vi "CRYGraph Property Window Result.vi"(8 "Tab Name":string, 9 "Graph VI Ref":refnum<vi>) -> ()   [LabVIEW 2013]
uses:
  Control/CRYResult Property.ctl
panel:
  in  "Redraw":bool
  in  "Draw":bool
  in  "Result Property":T1={"Show Limits"=FALSE, "Show Yield"=FALSE, "Pass/Fail"=FALSE, "Notation"=0, "Digits"=0, "Precision"=0, "Hide Traling Zeros"=FALSE, "Show vertical scroll bar"=FALSE, "Show horizontal scroll bar"=FALSE, "True"="NO ELECTRICAL SIGNAL DETECTED!\nCheck wiring and connections.", "False"="NO ELECTRICAL SIGNAL DETECTED!\nCheck wiring and connections.", "Font Size"=0, "Overall/Optional"=0} {"Precision" items=["Digits of precision", "Significant digits"]}
  in  "OK":bool
  in  "Result Tab":enum32{"Title", "Format"}(tab)
  in  "Title Name":string
  in  "Show vertical scroll bar":bool
  in  "Show horizontal scroll bar":bool
  in  "Overall/Optional":u16(slide) caption="Notation"
  in  "Font Size":u16
  in  "False":string
  in  "True":string
  in  "Hide Traling Zeros":bool caption="Hide Trailing Zeros"
  in  "PrecisionType":u16(ring) caption="Precision" items=["Digitals of precision", "Significant digits "]
  in  "Digits":u16
  in  "Notation":u16(slide)
  in  "Pass/Fail":bool
  in  "Show Yield":bool
  in  "Show Limits":bool
  out "Number Format":bool
  out "Settings":bool
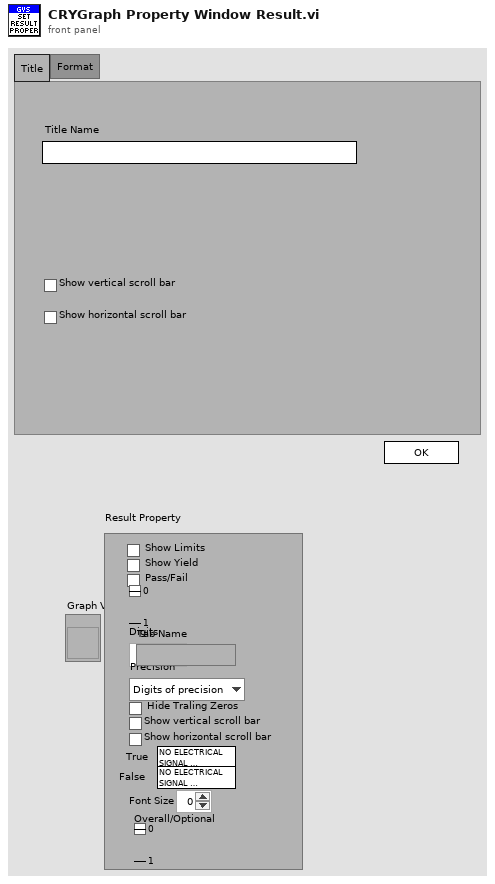
[diagram p1: front panel]
types:
  T1 = typedef "CRYResult Property.ctl" = cluster{"Show Limits":bool, "Show Yield":bool, "Pass/Fail":bool, "Notation":u16, "Digits":u16, "Precision":u16, "Hide Traling Zeros":bool, "Show vertical scroll bar":bool, "Show horizontal scroll bar":bool, "True":string, "False":string, "Font Size":u16, "Overall/Optional":u16}
  T2 = enum32{"Page Enabled", "Page Disabled", "Page Disabled & Grayed"}
  T3 = enum8{"Enabled", "Disabled", "Disabled and Grayed Out"}
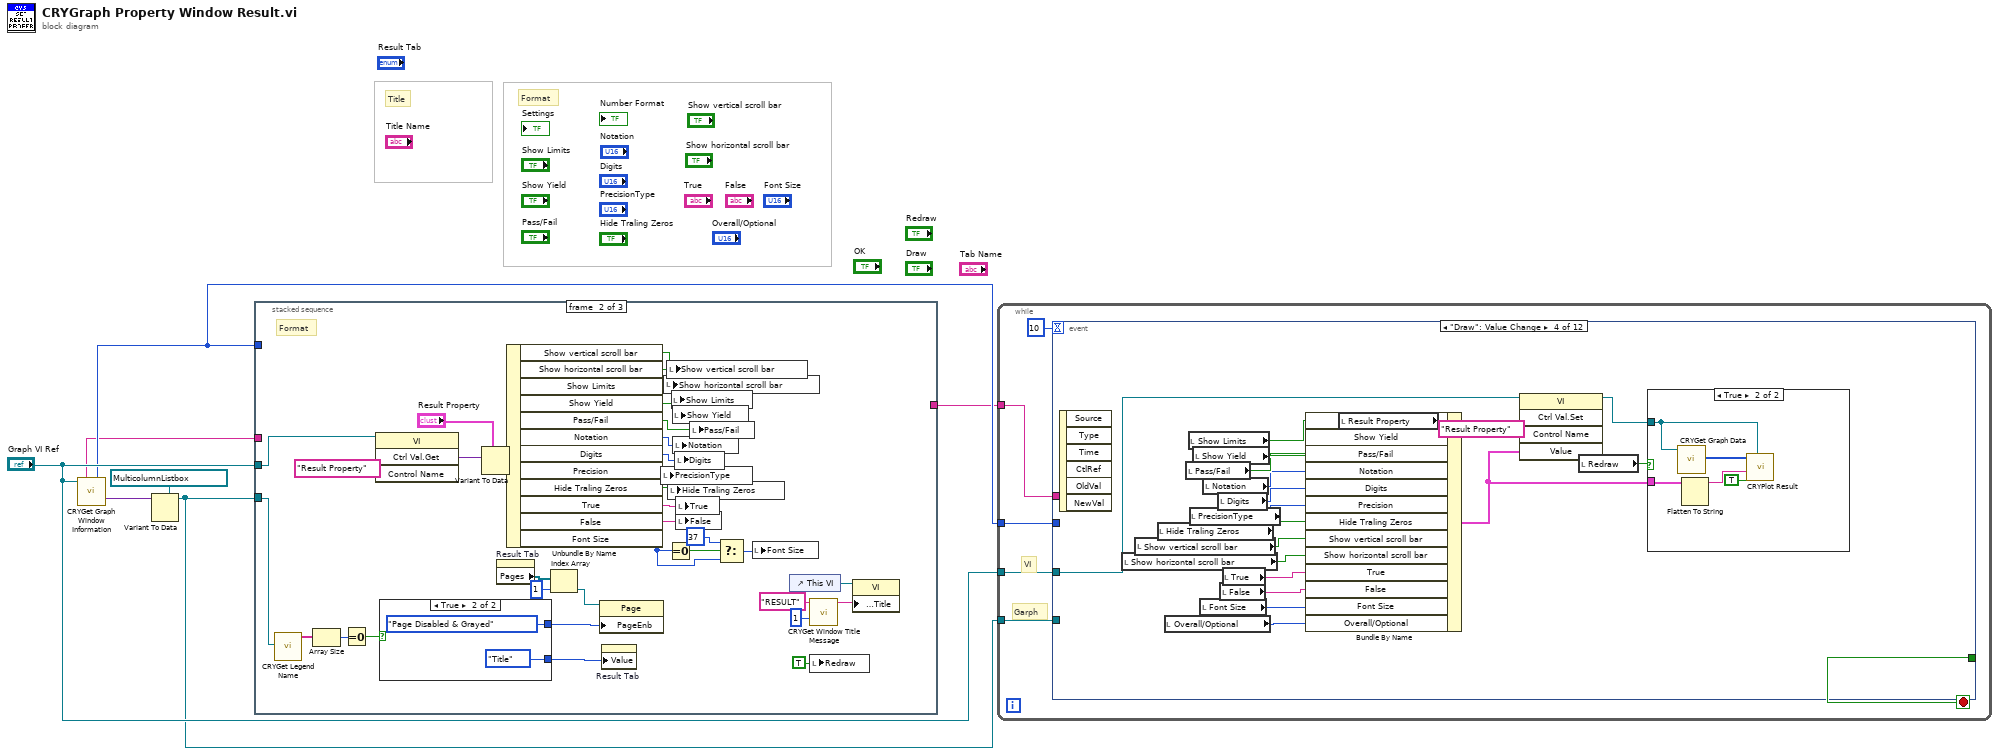
[diagram p0: block diagram]
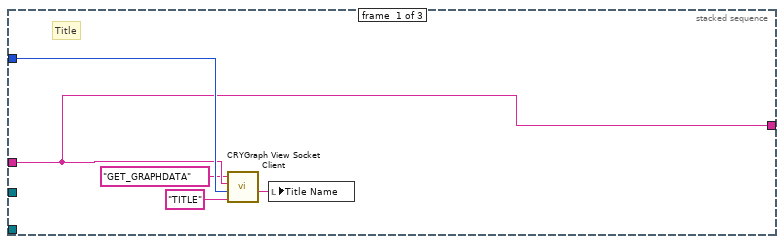
[diagram p2: hidden frame]
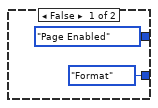
[diagram p3: hidden frame]
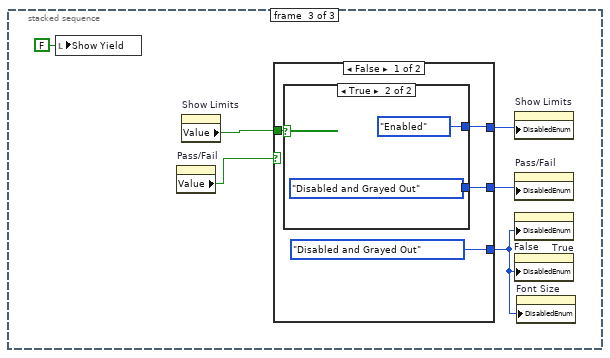
[diagram p4: hidden frame]
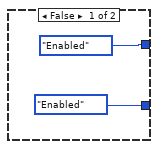
[diagram p5: hidden frame]
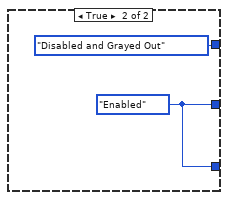
[diagram p6: hidden frame]
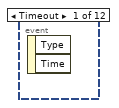
[diagram p7: hidden frame]
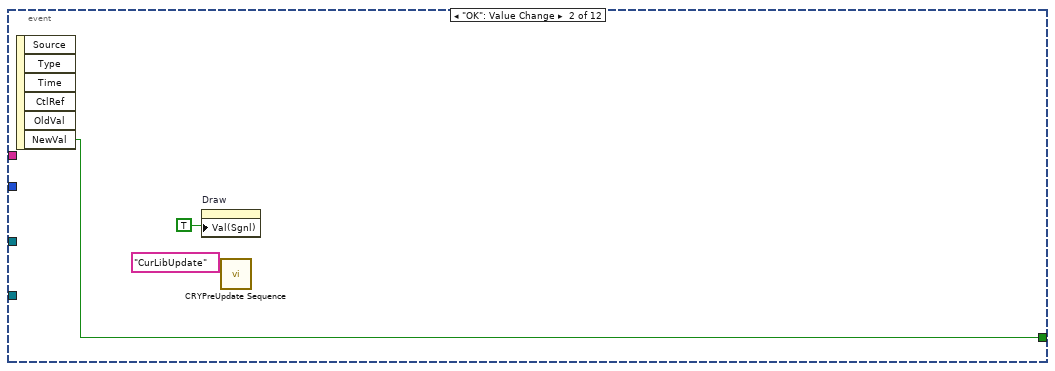
[diagram p8: hidden frame]
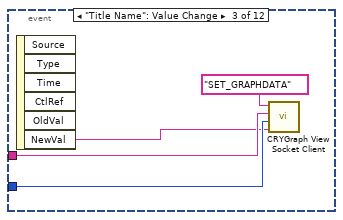
[diagram p9: hidden frame]
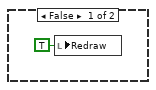
[diagram p10: hidden frame]
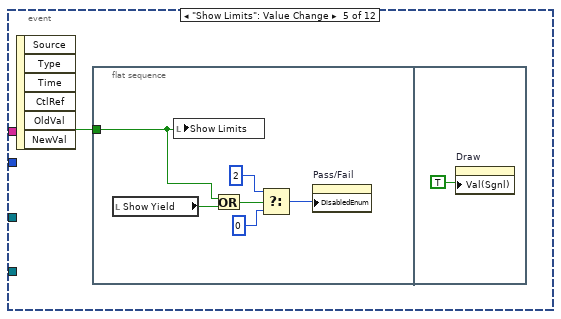
[diagram p11: hidden frame]
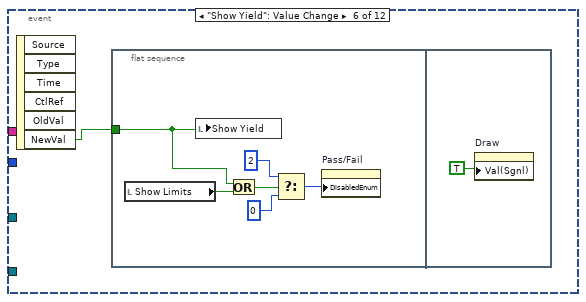
[diagram p12: hidden frame]
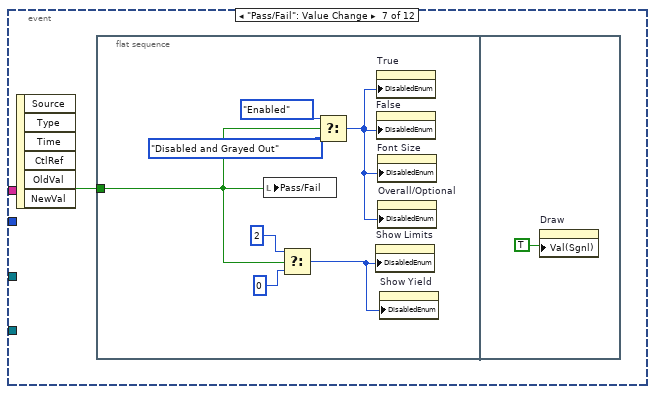
[diagram p13: hidden frame]
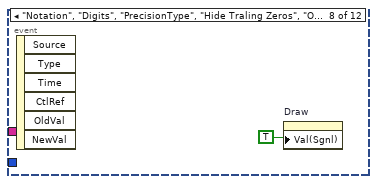
[diagram p14: hidden frame]
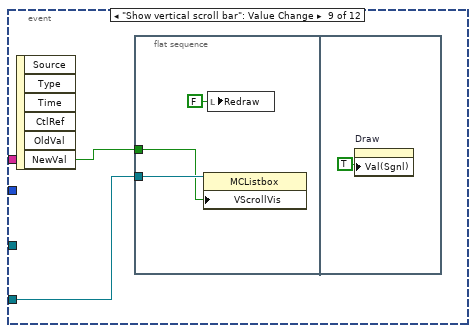
[diagram p15: hidden frame]
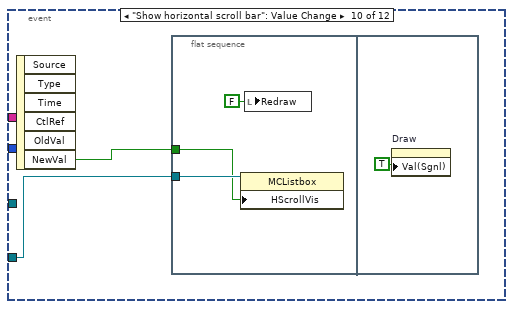
[diagram p16: hidden frame]
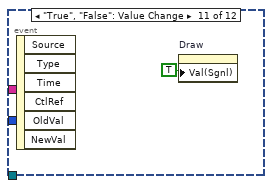
[diagram p17: hidden frame]
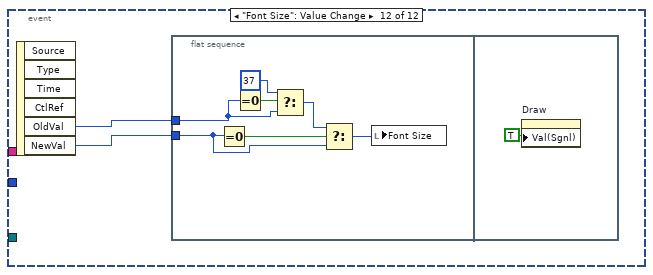
[diagram p18: hidden frame]
diagram:
  # "Title"
  # "Format"
  n1 = call "CRYGet Graph Window Information.vi"("pGraph VI In"="Graph VI Ref") -> ("Queue Name Out"=w4:string, "Graph Number Out"=w5:i32, "Graph Control Ref Out"=w1:variant)  [unwired: 2 in, 10 out]
  n2 = Variant To Data(type=refnum<vi> refnum ("Graph Ref"), Variant=w1) -> (data=w6:refnum<vi>)  [unwired: 1 in, 1 out]
  n3 = stacked-sequence {
    tunnel: "Graph VI Ref" -> [_ w46 _]
    tunnel: w6 -> [_ w28 _]
    tunnel: w5 -> [w12 _ _]
    tunnel: w4 -> [w11 _ _]
    tunnel: [w11 _ _] -> w3
    frame #0 {
      # "Title"
      n4 = call "CRYGraph View Socket Client.vi"("sOption"="TITLE", "nData"=w12, "sData"=w11, "sAction"="GET_GRAPHDATA") -> ("sData Out"=w8:string)  [unwired: 4 in, 3 out]
      n5 = local write "Title Name"(w8) -> ()
    }
    frame #1 {
      # "Format"
      n6 = call "CRYGet Legend Name.vi"("MCListbox Refnum"=w28) -> ("Names Out"=w36:string[])  [unwired: 1 in, 9 out]
      n7 = Array Size(array=w36) -> (size(s)=w35:i32)
      n8 = Equal To 0?(x=w35) -> (x = 0?=w32:bool)
      n9 = invoke class="VI" method="Ctrl Val.Get"(reference=w46, "Control Name"="Result Property") -> ("Get Control Value Variant"=w44:variant)  [unwired: 2 in, 3 out]
      n10 = case shown="True" w32 {
        tunnel: [T2."Page Enabled" ("Page Enabled State") T2."Page Disabled & Grayed" ("Page Enabled State")] -> w30
        tunnel: [enum32{"Title", "Format"}."Format" ("Tab Control") enum32{"Title", "Format"}."Title" ("Tab Control")] -> w29
        frame False {
        }
        frame True {
        }
      }
      n11 = Variant To Data(type="Result Property", Variant=w44) -> (data=w43:T1)  [unwired: 1 in, 1 out]
      n12 = property on="Result Tab" class="TabCtl (strict)"() -> ("Pages"=w34:refnum<vi>[])  [unwired: 2 in, 2 out]
      n13 = Unbundle By Name(w43) -> ("Show vertical scroll bar"=w20:bool, "Show horizontal scroll bar"=w19:bool, "Show Limits"=w23:bool, "Show Yield"=w42:bool, "Pass/Fail"=w41:bool, "Notation"=w40:u16, "Digits"=w39:u16, "Precision"=w38:u16, "Hide Traling Zeros"=w37:bool, "True"=w18:string, "False"=w17:string, "Font Size"=w14:u16)
      n14 = Index Array(array=w34, index=1) -> (element=w31:refnum<vi>)
      n15 = property class="Page"(reference=w31, "PageEnb"=w30) -> ()  [unwired: 1 in, 2 out]
      n16 = property on="Result Tab" class="TabCtl (strict)"("Value"=w29) -> ()  [unwired: 2 in, 2 out]
      n17 = local write "PrecisionType"(w38) -> ()
      n18 = local write "Show horizontal scroll bar"(w19) -> ()
      n19 = local write "Show vertical scroll bar"(w20) -> ()
      n20 = Equal To 0?(x=w14) -> (x = 0?=w15:bool)
      n21 = local write "Hide Traling Zeros"(w37) -> ()
      n22 = local write "Show Limits"(w23) -> ()
      n23 = local write "Show Yield"(w42) -> ()
      n24 = local write "Notation"(w40) -> ()
      n25 = local write "Digits"(w39) -> ()
      n26 = local write "True"(w18) -> ()
      n27 = local write "False"(w17) -> ()
      n28 = local write "Pass/Fail"(w41) -> ()
      n29 = Select(t=u16 37, s=w15, f=w14) -> (s? t:f=w13:u16)
      n30 = local write "Font Size"(w13) -> ()
      n31 = control-ref of="This VI"() -> (w24:refnum<vi>)
      n32 = call "CRYGet Window Title Message.vi"("No"=1 ("Error No"), "Kind"="RESULT") -> ("Multibyte String"=w25:string)  [unwired: 4 in, 5 out]
      n33 = local write "Redraw"(TRUE ("Redraw")) -> ()
      n34 = property class="VI"(reference=w24, "Front Panel.Title"=w25) -> ()  [unwired: 1 in, 2 out]
    }
    frame #2 {
      n35 = local write "Show Yield"(FALSE ("Show Yield")) -> ()
      n36 = property on="Pass/Fail" class="Bool (strict)"() -> ("Value"=w53:bool)  [unwired: 2 in, 2 out]
      n37 = property on="Show Limits" class="Bool (strict)"() -> ("Value"=w55:bool)  [unwired: 2 in, 2 out]
      n38 = case shown="False" w53 {
        tunnel: [w58 w65] -> w52
        tunnel: [w59 T3."Disabled and Grayed Out" ("Disabled")] -> w54
        tunnel: w55 -> [w60 _]
        tunnel: [T3."Disabled and Grayed Out" ("Disabled") w65] -> w51
        frame False {
          n39 = case shown="True" w60 {
            tunnel: [T3."Enabled" ("Disabled") T3."Enabled" ("Disabled")] -> w59
            tunnel: [T3."Enabled" ("Disabled") T3."Disabled and Grayed Out" ("Disabled")] -> w58
            frame False {
            }
            frame True {
            }
          }
        }
        frame True {
          w65 = T3."Enabled" ("Disabled")
        }
      }
      n40 = property on="Show Limits" class="Bool (strict)"("DisabledEnum"=w54) -> ()  [unwired: 2 in, 2 out]
      n41 = property on="Pass/Fail" class="Bool (strict)"("DisabledEnum"=w52) -> ()  [unwired: 2 in, 2 out]
      n42 = property on="True" class="Str"("DisabledEnum"=w51) -> ()  [unwired: 2 in, 2 out]
      n43 = property on="False" class="Str"("DisabledEnum"=w51) -> ()  [unwired: 2 in, 2 out]
      n44 = property on="Font Size" class="DigNum (strict)"("DisabledEnum"=w51) -> ()  [unwired: 2 in, 2 out]
    }
  }
  n45 = while {
    tunnel: w5 -> [w71]
    tunnel: "Graph VI Ref" -> [w70]
    tunnel: w6 -> [w69]
    tunnel: w3 -> [w67]
    stop <- w68 stop-if-true
    # "Garph"
    # "VI"
    n46 = event shown="[3] \"Draw\": Value Change" {
      selector: _ -> [_ _ _ _ _ _ _ _ _ _ _ _]
      dyn-events: _ -> [_ _ _ _ _ _ _ _ _ _ _ _]
      timeout: 10 -> [_ _ _ _ _ _ _ _ _ _ _ _]
      tunnel: [_ w75 _ _ _ _ _ _ _ _ _ _] -> w68
      tunnel: w71 -> [_ _ w78 _ _ _ _ _ _ _ _ _]
      tunnel: w70 -> [_ _ _ w98 _ _ _ _ _ _ _ _]
      tunnel: w69 -> [_ _ _ _ _ _ _ _ w132 w138 _ _]
      tunnel: w67 -> [_ _ w77 _ _ _ _ _ _ _ _ _]
      event Timeout {
        n47 = event-data() -> ()  [unwired: 3 out]
      }
      event "OK": Value Change {
        n48 = event-data() -> ("NewVal"=w75:bool)  [unwired: 6 out]
        n49 = property on="Draw" class="Bool (strict)"("Val(Sgnl)"=TRUE) -> ()  [unwired: 2 in, 2 out]
        n50 = call "CRYPreUpdate Sequence.vi"("EventName"="CurLibUpdate") -> ()  [unwired: 15 in]
      }
      event "Title Name": Value Change {
        n51 = event-data() -> ("NewVal"=w76:string)  [unwired: 6 out]
        n52 = call "CRYGraph View Socket Client.vi"("sOption"=w76, "nData"=w78, "sData"=w77, "sAction"="SET_GRAPHDATA") -> ()  [unwired: 4 in, 4 out]
      }
      event "Draw": Value Change {
        n53 = event-data() -> ()  [unwired: 7 out]
        n54 = local read "Show horizontal scroll bar"() -> (w84:bool)
        n55 = local read "Show vertical scroll bar"() -> (w85:bool)
        n56 = local read "Hide Traling Zeros"() -> (w87:bool)
        n57 = local read "Overall/Optional"() -> (w80:u16)
        n58 = local read "Pass/Fail"() -> (w91:bool)
        n59 = local read "Show Limits"() -> (w93:bool)
        n60 = local read "PrecisionType"() -> (w88:u16)
        n61 = local read "Show Yield"() -> (w92:bool)
        n62 = local read "Font Size"() -> (w81:u16)
        n63 = local read "Notation"() -> (w90:u16)
        n64 = local read "Digits"() -> (w89:u16)
        n65 = local read "False"() -> (w82:string)
        n66 = local read "True"() -> (w83:string)
        n67 = local read "Result Property"() -> (w94:T1)
        n68 = Bundle By Name(cluster=w94, "Show Limits"=w93, "Show Yield"=w92, "Pass/Fail"=w91, "Notation"=w90, "Digits"=w89, "Precision"=w88, "Hide Traling Zeros"=w87, "Show vertical scroll bar"=w85, "Show horizontal scroll bar"=w84, "True"=w83, "False"=w82, "Font Size"=w81, "Overall/Optional"=w80) -> (w97:T1)
        n69 = invoke class="VI" method="Ctrl Val.Set"(reference=w98, "Control Name"="Result Property", "Value"=w97) -> (reference out=w96:refnum<vi>)  [unwired: 2 in, 4 out]
        n70 = local read "Redraw"() -> (w86:bool)
        n71 = case shown="True" w86 {
          tunnel: w97 -> [_ w103]
          tunnel: w96 -> [_ w100]
          frame False {
            n72 = local write "Redraw"(TRUE ("Redraw")) -> ()
          }
          frame True {
            n73 = call "CRYGet Graph Data.vi"("pGraph VI"=w100) -> ("Rows"=w104:i32[])  [unwired: 2 in, 8 out]
            n74 = Flatten To String(anything=w103) -> (data string=w102:string)  [unwired: 3 in, 2 out]
            n75 = call "CRYPlot Result.vi"("pGraph VI In"=w100, "Graph Set?"=TRUE, "Flattened Property"=w102, "Old Rows In"=w104) -> ()  [unwired: 2 in, 6 out]
          }
        }
      }
      event "Show Limits": Value Change {
        n76 = event-data() -> ("NewVal"=w105:bool)  [unwired: 6 out]
        n77 = flat-sequence {
          tunnel: w105 -> [w110]
          frame #0 {
            n78 = local read "Show Yield"() -> (w111:bool)
            n79 = local write "Show Limits"(w110) -> ()
            n80 = Or(x=w110, y=w111) -> (x .or. y?=w109:bool)
            n81 = Select(t=2, s=w109, f=0) -> (s? t:f=w106:i32)
            n82 = property on="Pass/Fail" class="Bool (strict)"("DisabledEnum"=w106) -> ()  [unwired: 2 in, 2 out]
          }
          frame #1 {
            n83 = property on="Draw" class="Bool (strict)"("Val(Sgnl)"=TRUE) -> ()  [unwired: 2 in, 2 out]
          }
        }
      }
      event "Show Yield": Value Change {
        n84 = event-data() -> ("NewVal"=w113:bool)  [unwired: 6 out]
        n85 = flat-sequence {
          tunnel: w113 -> [w115]
          frame #0 {
            n86 = local read "Show Limits"() -> (w119:bool)
            n87 = local write "Show Yield"(w115) -> ()
            n88 = Or(x=w115, y=w119) -> (x .or. y?=w118:bool)
            n89 = Select(t=2, s=w118, f=0) -> (s? t:f=w114:i32)
            n90 = property on="Pass/Fail" class="Bool (strict)"("DisabledEnum"=w114) -> ()  [unwired: 2 in, 2 out]
          }
          frame #1 {
            n91 = property on="Draw" class="Bool (strict)"("Val(Sgnl)"=TRUE) -> ()  [unwired: 2 in, 2 out]
          }
        }
      }
      event "Pass/Fail": Value Change {
        n92 = event-data() -> ("NewVal"=w121:bool)  [unwired: 6 out]
        n93 = flat-sequence {
          tunnel: w121 -> [w125]
          frame #0 {
            n94 = local write "Pass/Fail"(w125) -> ()
            n95 = Select(t=2, s=w125, f=0) -> (s? t:f=w126:i32)
            n96 = Select(t=T3."Enabled" ("Disabled"), s=w125, f=T3."Disabled and Grayed Out" ("Disabled")) -> (s? t:f=w122:T3)
            n97 = property on="Show Limits" class="Bool (strict)"("DisabledEnum"=w126) -> ()  [unwired: 2 in, 2 out]
            n98 = property on="True" class="Str"("DisabledEnum"=w122) -> ()  [unwired: 2 in, 2 out]
            n99 = property on="False" class="Str"("DisabledEnum"=w122) -> ()  [unwired: 2 in, 2 out]
            n100 = property on="Font Size" class="DigNum (strict)"("DisabledEnum"=w122) -> ()  [unwired: 2 in, 2 out]
            n101 = property on="Overall/Optional" class="Slide (strict)"("DisabledEnum"=w122) -> ()  [unwired: 2 in, 2 out]
            n102 = property on="Show Yield" class="Bool (strict)"("DisabledEnum"=w126) -> ()  [unwired: 2 in, 2 out]
          }
          frame #1 {
            n103 = property on="Draw" class="Bool (strict)"("Val(Sgnl)"=TRUE) -> ()  [unwired: 2 in, 2 out]
          }
        }
      }
      event "Notation", "Digits", "PrecisionType", "Hide Traling Zeros", "Overall/Optional": Value Change {
        n104 = event-data() -> ()  [unwired: 7 out]
        n105 = property on="Draw" class="Bool (strict)"("Val(Sgnl)"=TRUE) -> ()  [unwired: 2 in, 2 out]
      }
      event "Show vertical scroll bar": Value Change {
        n106 = event-data() -> ("NewVal"=w131:bool)  [unwired: 6 out]
        n107 = flat-sequence {
          tunnel: w132 -> [w134]
          tunnel: w131 -> [w133]
          frame #0 {
            n108 = property class="MCListbox"(reference=w134, "VScrollVis"=w133) -> ()  [unwired: 1 in, 2 out]
            n109 = local write "Redraw"(FALSE ("Redraw")) -> ()
          }
          frame #1 {
            n110 = property on="Draw" class="Bool (strict)"("Val(Sgnl)"=TRUE) -> ()  [unwired: 2 in, 2 out]
          }
        }
      }
      event "Show horizontal scroll bar": Value Change {
        n111 = event-data() -> ("NewVal"=w137:bool)  [unwired: 6 out]
        n112 = flat-sequence {
          tunnel: w138 -> [w140]
          tunnel: w137 -> [w139]
          frame #0 {
            n113 = property class="MCListbox"(reference=w140, "HScrollVis"=w139) -> ()  [unwired: 1 in, 2 out]
            n114 = local write "Redraw"(FALSE ("Redraw")) -> ()
          }
          frame #1 {
            n115 = property on="Draw" class="Bool (strict)"("Val(Sgnl)"=TRUE) -> ()  [unwired: 2 in, 2 out]
          }
        }
      }
      event "True", "False": Value Change {
        n116 = event-data() -> ()  [unwired: 7 out]
        n117 = property on="Draw" class="Bool (strict)"("Val(Sgnl)"=TRUE) -> ()  [unwired: 2 in, 2 out]
      }
      event "Font Size": Value Change {
        n118 = event-data() -> ("OldVal"=w144:u16, "NewVal"=w145:u16)  [unwired: 5 out]
        n119 = flat-sequence {
          tunnel: w145 -> [w151]
          tunnel: w144 -> [w149]
          frame #0 {
            n120 = Equal To 0?(x=w151) -> (x = 0?=w152:bool)
            n121 = Equal To 0?(x=w149) -> (x = 0?=w150:bool)
            n122 = Select(t=u16 37, s=w150, f=w149) -> (s? t:f=w148:u16)
            n123 = Select(t=w148, s=w152, f=w151) -> (s? t:f=w146:u16)
            n124 = local write "Font Size"(w146) -> ()
          }
          frame #1 {
            n125 = property on="Draw" class="Bool (strict)"("Val(Sgnl)"=TRUE) -> ()  [unwired: 2 in, 2 out]
          }
        }
      }
    }
  }
